vi "RIGOLsweepsetup.vi"(8 "AP Sweep Width (MHz)":dbl, 9 "Time (ms)":dbl, 10 "Amplitude (Vpp)":dbl, 11 "Frequency (MHz)":dbl) -> ()   [LabVIEW 2012]
uses:
  <vilib>/Instr/_visa.llb/VISA Open Access Mode.ctl
panel:
  out "read buffer":string
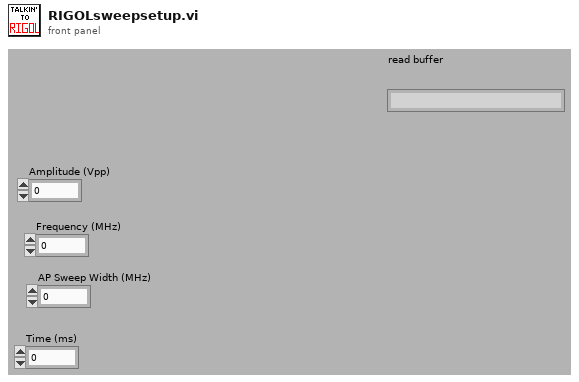
[diagram p1: front panel]
types:
  T1 = typedef "VISA Open Access Mode.ctl" = u32
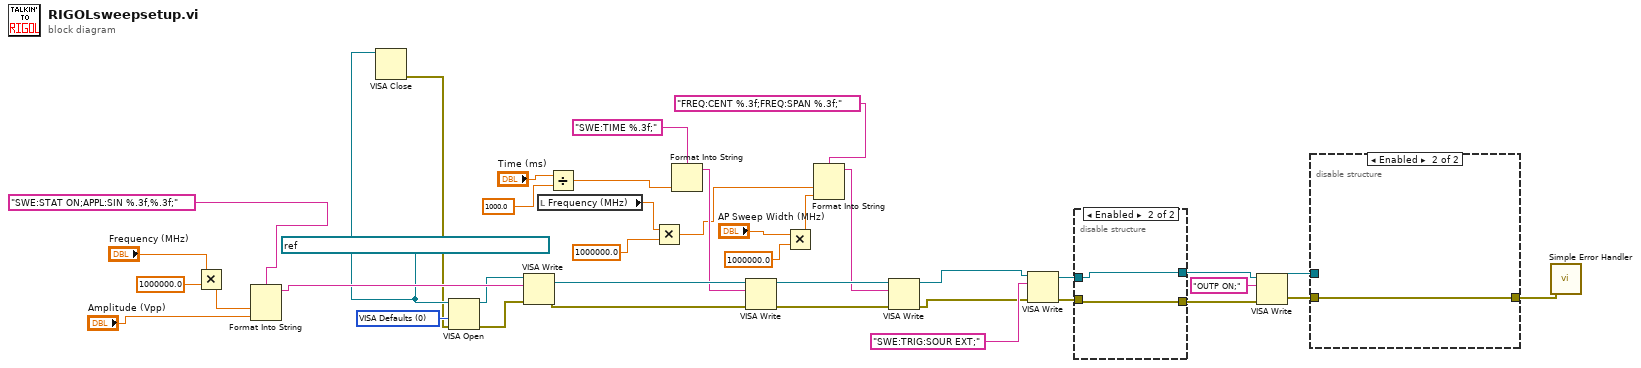
[diagram p0: block diagram]
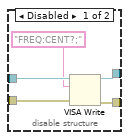
[diagram p2: hidden frame]
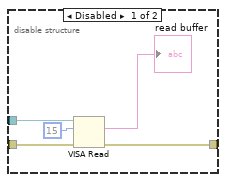
[diagram p3: hidden frame]
diagram:
  w3 = T1 0 items=["VISA Defaults"=0, "Exclusive Lock"=1, "Load Configured Settings"=4] ("Access Mode")
  w2 = refnum<visa-resource-name> "USB0::0x1AB1::0x0641::DG4B142100247::INSTR" ("VISA resource name")
  n1 = Multiply(x="Frequency (MHz)", y=1000000.0) -> (x*y=w37:dbl)
  n2 = Format Into String(format string="SWE:STAT ON;APPL:SIN %.3f,%.3f;", w37, "Amplitude (Vpp)") -> (resulting string=w8:string)  [unwired: 2 in, 1 out]
  n3 = VISA Close(VISA resource name=w2) -> (error out=w1:errorcluster)  [unwired: 1 in]
  n4 = VISA Open(access mode=w3, error in (no error)=w1, VISA resource name=w2) -> (VISA resource name=w5:refnum<visa-resource-name>, error out=w4:errorcluster)  [unwired: 2 in]
  n5 = VISA Write(VISA resource name=w5, write buffer=w8, error in (no error)=w4) -> (VISA resource name out=w35:refnum<visa-resource-name>, error out=w34:errorcluster)  [unwired: 1 out]
  n6 = local read "Frequency (MHz)"() -> (w16:dbl)
  n7 = Divide(x="Time (ms)", y=1000.0) -> (x/y=w19:dbl)
  n8 = Multiply(x=w16, y=1000000.0) -> (x*y=w6:dbl)
  n9 = Format Into String(format string="SWE:TIME %.3f;" ("write buffer"), w19) -> (resulting string=w10:string)  [unwired: 2 in, 1 out]
  n10 = VISA Write(VISA resource name=w35, write buffer=w10, error in (no error)=w34) -> (VISA resource name out=w33:refnum<visa-resource-name>, error out=w32:errorcluster)  [unwired: 1 out]
  n11 = Multiply(x="AP Sweep Width (MHz)", y=1000000.0) -> (x*y=w7:dbl)
  n12 = Format Into String(format string="FREQ:CENT %.3f;FREQ:SPAN %.3f;" ("write buffer"), w6, w7) -> (resulting string=w15:string)  [unwired: 2 in, 1 out]
  n13 = VISA Write(VISA resource name=w33, write buffer=w15, error in (no error)=w32) -> (VISA resource name out=w26:refnum<visa-resource-name>, error out=w25:errorcluster)  [unwired: 1 out]
  n14 = VISA Write(VISA resource name=w26, write buffer="SWE:TRIG:SOUR EXT;", error in (no error)=w25) -> (VISA resource name out=w21:refnum<visa-resource-name>, error out=w20:errorcluster)  [unwired: 1 out]
  n15 = disable-structure shown="Enabled" {
    disable-tunnel: [w44 w46] -> w23
    disable-tunnel: [w43 w45] -> w22
    disable-tunnel: w21 -> [w42 w46]
    disable-tunnel: w20 -> [w41 w45]
    frame Disabled {
      n16 = VISA Write(VISA resource name=w42, write buffer="FREQ:CENT?;", error in (no error)=w41) -> (VISA resource name out=w44:refnum<visa-resource-name>, error out=w43:errorcluster)  [unwired: 1 out]
    }
    frame Enabled {
    }
  }
  n17 = VISA Write(VISA resource name=w23, write buffer="OUTP ON;", error in (no error)=w22) -> (VISA resource name out=w29:refnum<visa-resource-name>, error out=w28:errorcluster)  [unwired: 1 out]
  n18 = disable-structure shown="Enabled" {
    disable-tunnel: w29 -> [w51 _]
    disable-tunnel: w28 -> [w50 w52]
    disable-tunnel: [w49 w52] -> w24
    frame Disabled {
      n19 = VISA Read(VISA resource name=w51, byte count=u32 15, error in (no error)=w50) -> (read buffer=→"read buffer":string, error out=w49:errorcluster)  [unwired: 2 out]
    }
    frame Enabled {
    }
  }
  n20 = call <vilib>:"Simple Error Handler.vi"("error in (no error)"=w24) -> ()  [unwired: 4 in, 5 out]
